vi "update.vi"(8 "error in (no error)":errorcluster, 11 "TrajectoryAK101022Resonance in":refnum<class "TrajectoryAK101022Resonance.lvclass">) -> (0 "error out":errorcluster, 3 "TrajectoryAK101022Resonance out":refnum<class "TrajectoryAK101022Resonance.lvclass">)   [LabVIEW 2010, in "TrajectoryAK101022Resonance.lvclass"]
uses:
  TrajectoryAK101022Resonance.lvclass
  FPGAWrapper/FPGAWrapperAK101022Resonance/scan_specification_cluster.ctl
  TrajectoryAK101022Resonance.lvclass/TrajectoryAK101022Resonance.ctl
  common/classes/GenericComponent/GenericComponent/class_data.vi
  common/classes/GenericComponent/GenericComponent/GenericComponent.lvclass
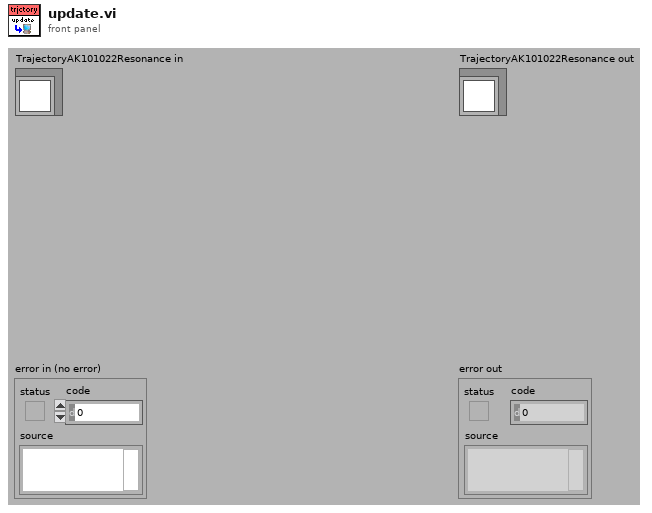
[diagram p1: front panel]
types:
  T1 = typedef "scan_specification_cluster.ctl" = cluster{"x amplitude":u16, "x resolution (pixels)":u16, "x offset fly-forward (iterations)":u16, "x offset fly-back (iterations)":u16, "y resolution (nr. of lines)":u16, "y step size":u16, "iterations per pixel":u16, "number of frames":i32, "y offset (pixels)":u16, "number of y-brake lines  (before y-fly-back)":u16, "number y-brake lines (after y-fly-back)":u16, "number of y-fly-back steps":u16, "lines per z step":u16, "number of z/intensity tuples":u16}
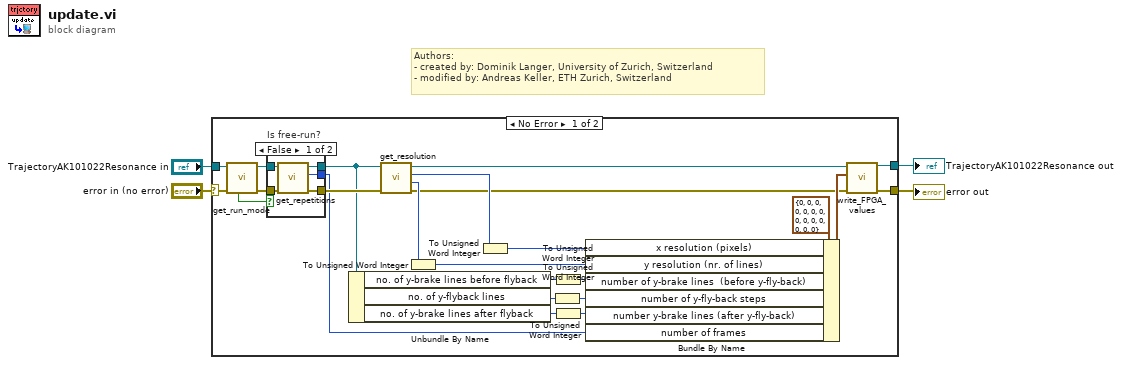
[diagram p0: block diagram]
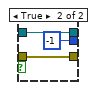
[diagram p2: hidden frame]
diagram:
  # "Authors: \n- created by: Dominik Langer, University of Zurich, Switzerland\n- modified by: Andreas Keller, ETH Zurich, Switzerland"
  n1 = case shown="No Error" "error in (no error)" {
    selector: "error in (no error)" -> [w9 w38]
    tunnel: "TrajectoryAK101022Resonance in" -> [w11 w37]
    tunnel: [w16 w38] -> w2
    tunnel: [w15 w37] -> w1
    frame No Error {
      n2 = call "get_run_mode.vi"("error in (no error)"=w9, "GenericPlugin in"=w11) -> ("error out"=w8:errorcluster, "GenericPlugin out"=w10:refnum<class "TrajectoryAK101022Resonance.lvclass">, "is free run?"=w7:bool)  [unwired: 5 in, 2 out]
      n3 = case "Is free-run?" shown="False" w7 {
        tunnel: [w33 w35] -> w26
        tunnel: [w32 -1 ("repetitions")] -> w6
        tunnel: [w31 w34] -> w17
        tunnel: w10 -> [w30 w34]
        tunnel: w8 -> [w29 w35]
        frame False {
          n4 = call-dynamic "get_repetitions.vi"("error in (no error)"=w29, "GenericTrajectory in"=w30) -> ("error out"=w33:errorcluster, "repetitions"=w32:i32, "GenericTrajectory out"=w31:refnum<class "TrajectoryAK101022Resonance.lvclass">)  [unwired: 7 in]
        }
        frame True {
        }
      }
      n5 = Unbundle By Name(w17) -> ("no. of y-brake lines before flyback"=w23:i32, "no. of y-flyback lines"=w22:i32, "no. of y-brake lines after flyback"=w21:i32)
      n6 = call-dynamic "get_resolution.vi"("error in (no error)"=w26, "TrajectoryAK101022Resonance in"=w17) -> ("error out"=w13:errorcluster, "y resolution"=w27:i32, "x resolution"=w25:i32, "TrajectoryAK101022Resonance out"=w12:refnum<class "TrajectoryAK101022Resonance.lvclass">)  [unwired: 6 in]
      n7 = To Unsigned Word Integer(number=w27) -> (unsigned 16bit integer=w28:u16)
      n8 = To Unsigned Word Integer(number=w25) -> (unsigned 16bit integer=w24:u16)
      n9 = To Unsigned Word Integer(number=w22) -> (unsigned 16bit integer=w19:u16)
      n10 = To Unsigned Word Integer(number=w23) -> (unsigned 16bit integer=w18:u16)
      n11 = To Unsigned Word Integer(number=w21) -> (unsigned 16bit integer=w20:u16)
      n12 = Bundle By Name(cluster=T1 {"x amplitude"=0, "x resolution (pixels)"=0, "x offset fly-forward (iterations)"=0, "x offset fly-back (iterations)"=0, "y resolution (nr. of lines)"=0, "y step size"=0, "iterations per pixel"=0, "number of frames"=0, "y offset (pixels)"=0, "number of y-brake lines  (before y-fly-back)"=0, "number y-brake lines (after y-fly-back)"=0, "number of y-fly-back steps"=0, "lines per z step"=0, "number of z/intensity tuples"=0} ("scan specification"), "x resolution (pixels)"=w24, "y resolution (nr. of lines)"=w28, "number of y-brake lines  (before y-fly-back)"=w18, "number of y-fly-back steps"=w19, "number y-brake lines (after y-fly-back)"=w20, "number of frames"=w6) -> (w14:T1)
      n13 = call-dynamic "write_FPGA_values.vi"("error in (no error)"=w13, "scan specification"=w14, "TrajectoryAK101022Resonance in"=w12) -> ("error out"=w16:errorcluster, "TrajectoryAK101022Resonance out"=w15:refnum<class "TrajectoryAK101022Resonance.lvclass">)  [unwired: 7 in]
    }
    frame Error {
    }
  }
  "error out" <- w2
  "TrajectoryAK101022Resonance out" <- w1
